vi "Update Staff Allocation.vi"(0 "Hotel Management Tool Model in":refnum<class "Hotel Management Tool Model.lvclass">, 5 "Staff Name":string[](array[string]), 7 "Service ID":string[](array[string]), 11 "error in (no error)":errorcluster) -> (4 "Hotel Management Tool Model out":refnum<class "Hotel Management Tool Model.lvclass">, 15 "error out":errorcluster)   [LabVIEW 2023, in "Hotel Management Tool Model.lvlib" / "Hotel Management Tool Model.lvclass"]
uses:
  Hotel Management Tool Model.lvclass
  Hotel Management Tool Model.lvclass/Hotel Management Tool Model.ctl
  Central Data Manager/Central Data Manager Messages/Update Staff Allocation Msg/Update Staff Allocation Msg.lvclass
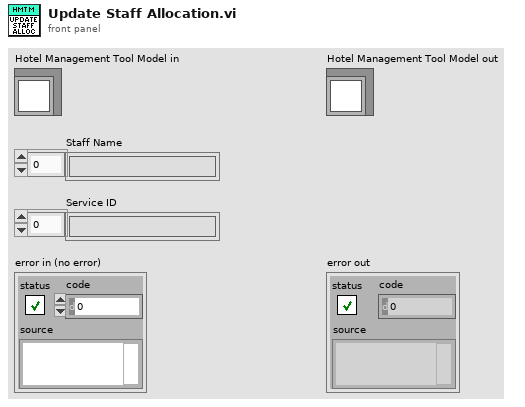
[diagram p1: front panel]
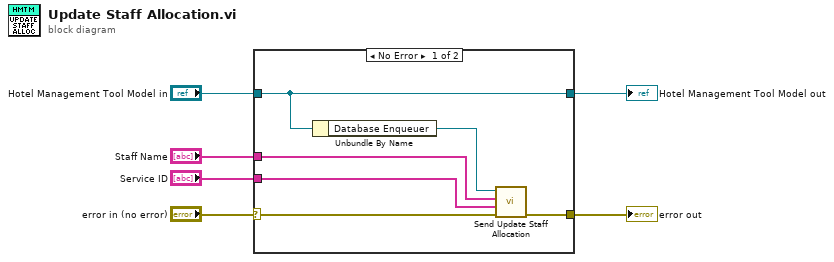
[diagram p0: block diagram]
diagram:
  n1 = case shown="No Error" "error in (no error)" {
    selector: "error in (no error)" -> [w12 w13]
    tunnel: "Hotel Management Tool Model in" -> [w11 w14]
    tunnel: [w11 w14] -> w5
    tunnel: [w10 w13] -> w4
    tunnel: "Staff Name" -> [w8 _]
    tunnel: "Service ID" -> [w7 _]
    frame No Error {
      n2 = Unbundle By Name(w11) -> ("Database Enqueuer"=w9:refnum<class "Message Enqueuer.lvclass">)
      n3 = call "Send Update Staff Allocation.vi"("error in (no error)"=w12, "Service ID"=w7, "Staff Name"=w8, "Message Enqueuer"=w9) -> ("error out"=w10:errorcluster)  [unwired: 6 in, 1 out]
    }
    frame Error {
    }
  }
  "error out" <- w4
  "Hotel Management Tool Model out" <- w5
